vi "Example.vi"() -> ()   [LabVIEW 2009]
panel:
  in  "Key Array":T1(array[cluster])=[{" Key"=16, "Action"=enum."Down", "Delay (ms)"=10}, {" Key"=72, "Action"=enum."Press", "Delay (ms)"=100}, {" Key"=16, "Action"=enum."Up", "Delay (ms)"=10}, {" Key"=69, "Action"=enum."Press", "Delay (ms)"=100}, {" Key"=76, "Action"=enum."Press", "Delay (ms)"=100}, {" Key"=76, "Action"=enum."Press", "Delay (ms)"=100}, {" Key"=79, "Action"=enum."Press", "Delay (ms)"=100}]
  in  "Output":string
  # "This VI is an example that uses simulated Key Presses to \ntype into a String control programmatically.  They Key Array \ncontrol is what defines which keys are pressed and for how\nlong.  Note that the shift key is pushed down and up in \nseparate steps and that the alphabetical keys are pressed.\nThis is equivalent to holding the shift key down while pressing\n'H', the result being an uppercase 'H'.\n\nSimply run this VI and 'Hello' will be programmatically typed in\nthe above Output box."
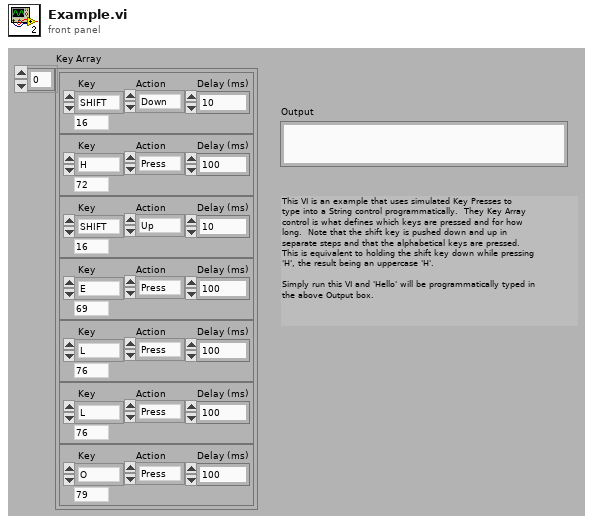
[diagram p1: front panel]
types:
  T1 = cluster{" Key":u8, "Action":enum16{"Press", "Up", "Down"}, "Delay (ms)":u32}[]
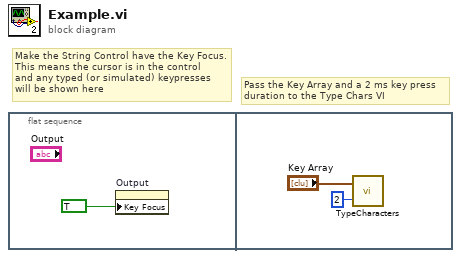
[diagram p0: block diagram]
diagram:
  # "Pass the Key Array and a 2 ms key press\nduration to the Type Chars VI"
  # "Make the String Control have the Key Focus.\nThis means the cursor is in the control\nand any typed (or simulated) keypresses\nwill be shown here"
  n1 = flat-sequence {
    frame #0 {
      n2 = property on="Output" class="Str"("Key Focus"=TRUE) -> ()  [unwired: 2 in, 2 out]
    }
    frame #1 {
      n3 = call "TypeCharacters.vi"("Length of Key Press (ms)"=u32 2, "Key Array"="Key Array") -> ()  [unwired: 1 in]
    }
  }
